vi "AllUnreserved.vi"() -> (3 "Pass?":bool)   [LabVIEW 2014]
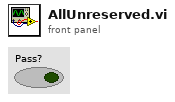
[diagram p1: front panel]
types:
  T1 = enum32{"Bad", "Idle", "Run top level", "Running"}
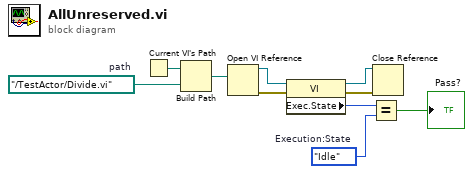
[diagram p0: block diagram]
diagram:
  w5 = T1."Idle"  # Execution:State
  w9 = path "../TestActor/Divide.vi"  # path
  n1 = Current VI's Path() -> (path=w10:path)
  n2 = Build Path(base path=w10, name or relative path=w9) -> (appended path=w8:path)
  n3 = Open VI Reference(vi path=w8) -> (vi reference=w7:refnum<vi>, error out=w4:errorcluster)  [unwired: 5 in]
  n4 = property class="VI"(reference=w7, error in=w4) -> (reference out=w3:refnum<vi>, error out=w2:errorcluster, "Exec.State"=w6:T1)
  n5 = Equal?(x=w6, y=w5) -> (x = y?=→"Pass?":bool)
  n6 = Close Reference(reference=w3, error in (no error)=w2) -> ()  [unwired: 1 out]
